vi "Config - Fire Event.vi"(8 "error in (no error)":errorcluster, 9 "DB Data":variant, 10 "DB Command":T1, 11 "View Model":T2) -> (0 "error out":errorcluster, 3 "View Model":T2)   [LabVIEW 2017]
doc: "Generate Config User Event from Controller."
uses:
  Model/Controls/View Model.ctl
  Model/Controls/Shared Model.ctl
  Error Handler/Controls/Error Model.ctl
  Error Handler/Controls/Error Message.ctl
  Error Handler/Controls/Error Type.ctl
  Controls/Config Model.ctl
  Controls/Config DB Message.ctl
  Controls/Config DB Command.ctl
  Controls/Config DB Overhead.ctl
  Controls/Config DB Record1.ctl
  Controls/Config DB Record2.ctl
  Controller/Controls/Controller Wash Step.ctl
  Views/Vehicle Position Simulation View/Controls/Vehicle - Position.ctl
  Controller/Controls/Controller Model.ctl
  Controller/Controls/Controller Overhead.ctl
  Controller/Controls/Controller State.ctl
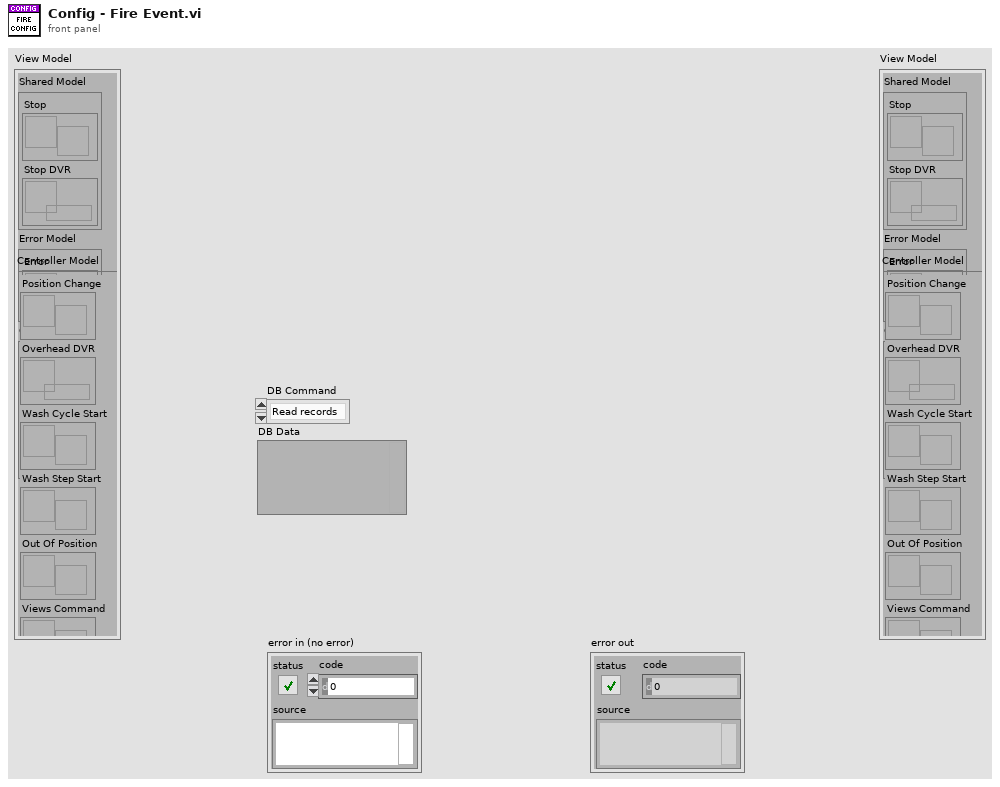
[diagram p1: front panel]
types:
  T1 = typedef "Config DB Command.ctl" = enum16{"Read records", "Query timing", "Insert new data", "Update data", "Lock DB", "Unlock DB"}
  T2 = typedef "View Model.ctl" = cluster{"Shared Model":T3, "Error Model":T4, "Config Model":T5, "Controller Model":T6}
  T3 = typedef "Shared Model.ctl" = cluster{"Stop":refnum<user-event>, "Stop DVR":refnum<data-value>}
  T4 = typedef "Error Model.ctl" = cluster{"Error":refnum<user-event>}
  T5 = typedef "Config Model.ctl" = cluster{"Config":refnum<user-event>, "Config DVR":refnum<data-value>}
  T6 = typedef "Controller Model.ctl" = cluster{"Position Change":refnum<user-event>, "Overhead DVR":refnum<data-value>, "Wash Cycle Start":refnum<user-event>, "Wash Step Start":refnum<user-event>, "Out Of Position":refnum<user-event>, "Views Command":refnum<user-event>}
  T7 = typedef "Config DB Message.ctl" = cluster{"DB Command":T1, "DB Data":variant}
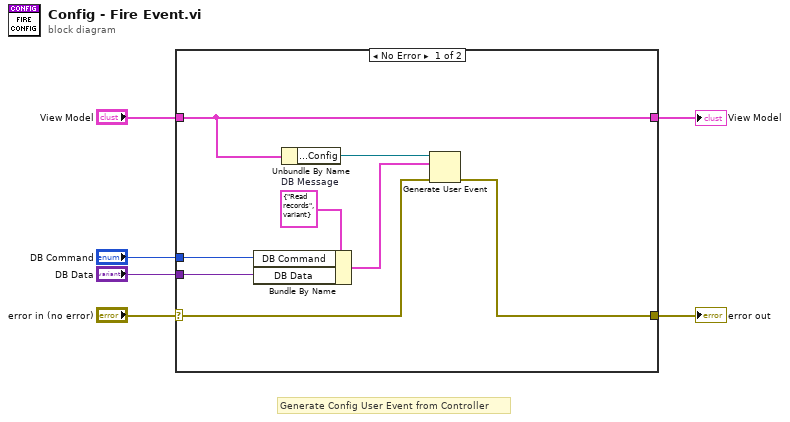
[diagram p0: block diagram]
diagram:
  # "Generate Config User Event from Controller"
  n1 = case shown="No Error" "error in (no error)" {
    selector: "error in (no error)" -> [w12 w16]
    tunnel: "View Model" -> [w13 w15]
    tunnel: [w11 w16] -> w4
    tunnel: [w13 w15] -> w3
    tunnel: "DB Data" -> [w8 _]
    tunnel: "DB Command" -> [w7 _]
    frame No Error {
      w10 = T7 {"DB Command"=enum."Read records", "DB Data"=variant}  # DB Message
      n2 = Bundle By Name(cluster=w10, "DB Command"=w7, "DB Data"=w8) -> (w9:T7)
      n3 = Unbundle By Name(w13) -> ("Config Model.Config"=w14:refnum<user-event>)
      n4 = Generate User Event(user event=w14, event data cluster=w9, error in=w12) -> (error out=w11:errorcluster)  [unwired: 1 in, 1 out]
    }
    frame Error {
    }
  }
  "View Model" <- w3
  "error out" <- w4
